vi "报警流程.vi"   [LabVIEW 2016, in "采配水.lvlib"]
uses:
  <vilib>/ptbypt/NI_PtbyPt.lvlib
types:
  T1 = cluster{"低压报警阈值 V":dbl, "低压报警解除阈值 V":dbl, "高温报警阈值 ℃":dbl, "高温报警解除阈值 ℃":dbl, "湿度报警阈值 %":dbl, "湿度报警解除阈值 %":dbl}
  T2 = cluster{"蓄电池电压":dbl, "室温":dbl, "湿度":dbl, "水浸报警":bool, "烟雾报警":bool, "门禁1状态":bool, "门禁2状态":bool}
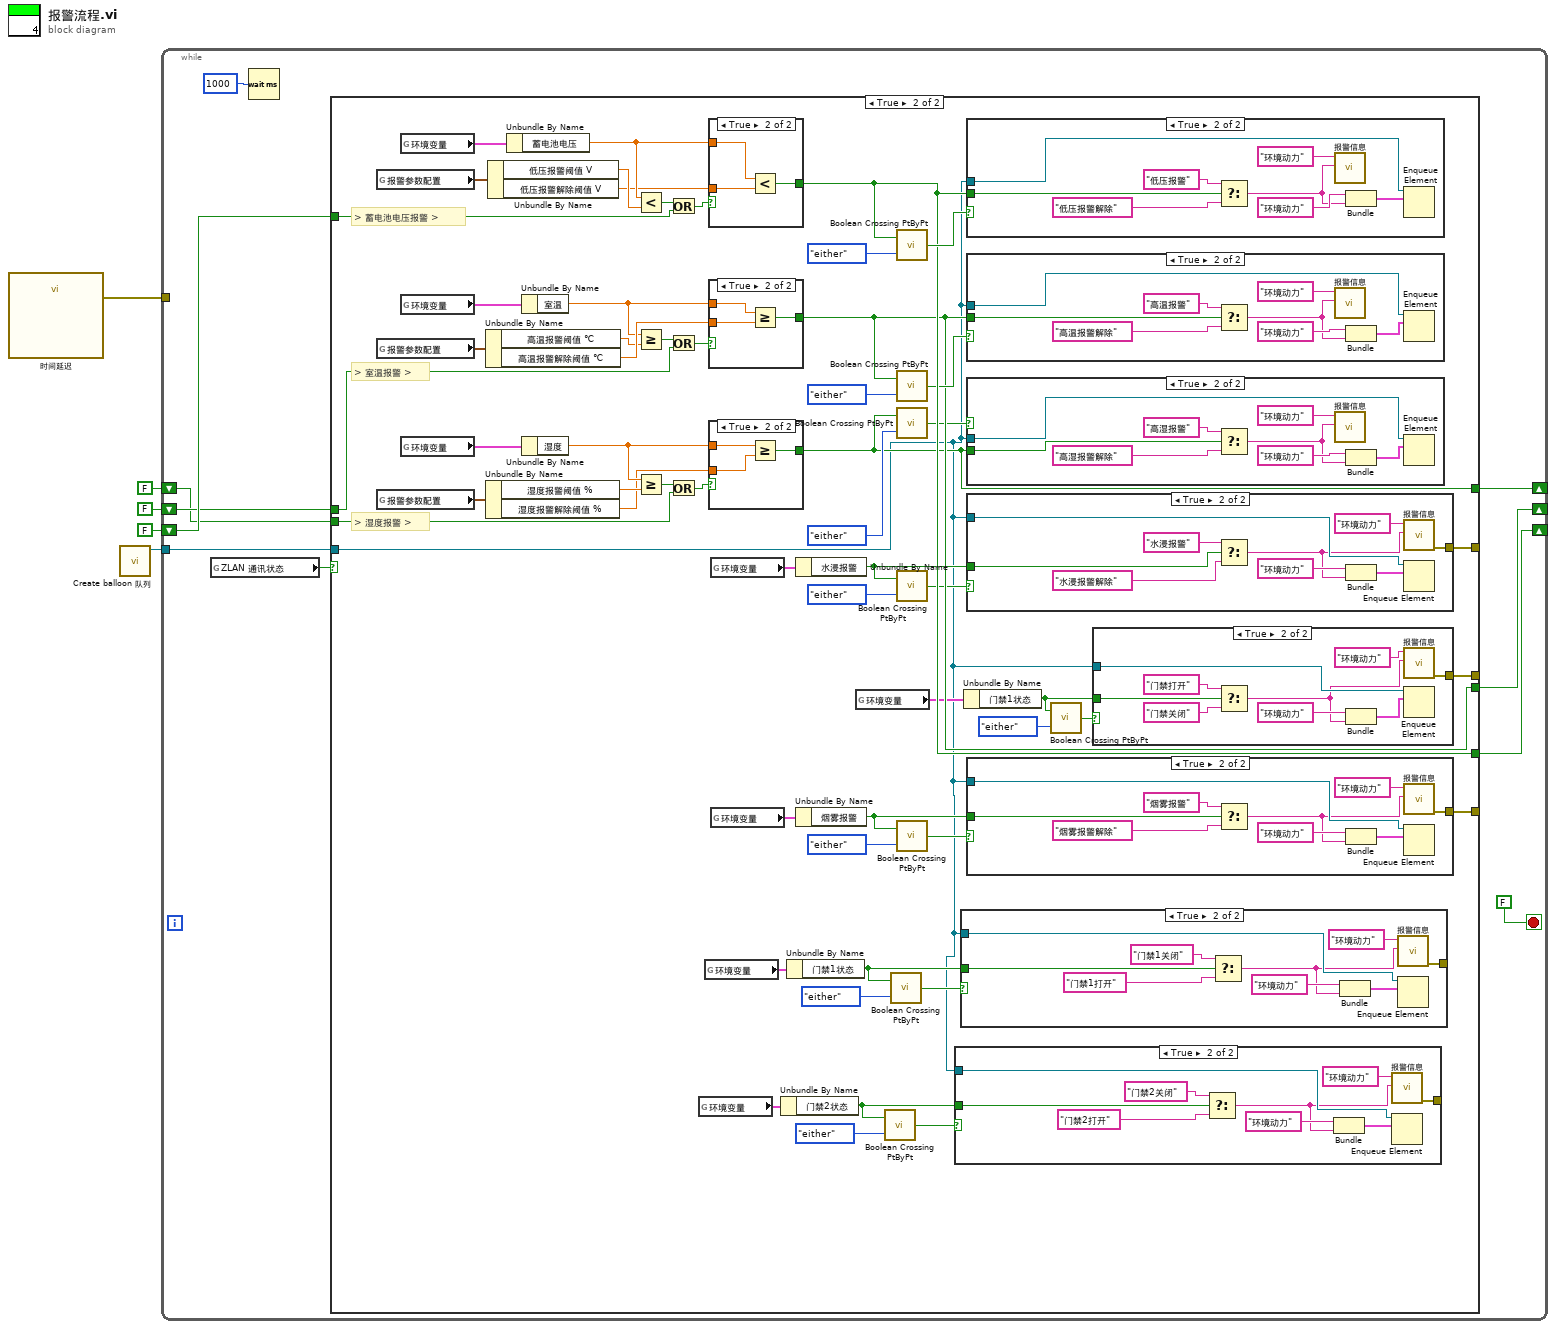
[diagram p0: block diagram]
diagram:
  n1 = call "时间延迟"() -> ("error out"=w1:errorcluster)  [unwired: 11 in]
  n2 = call "Create balloon 队列.vi"() -> ("队列输出"=w5:refnum<queue>)  [unwired: 11 in]
  n3 = while {
    shift-right: [w13] -> _
    shift-left: FALSE -> [w12]
    shift-right: [w10] -> _
    shift-left: FALSE -> [w11]
    shift-right: [w9] -> _
    shift-left: FALSE -> [w8]
    tunnel: w5 -> [w6]
    tunnel: w1 -> [_]
    stop <- FALSE stop-if-true
    n4 = global read "通讯全局变量.vi" "ZLAN 通讯状态"() -> (w7:bool)
    n5 = Wait (ms)(milliseconds to wait=u32 1000 ("等待时间（毫秒）")) -> ()  [unwired: 1 out]
    n6 = case shown="True" w7 {
      tunnel: [_ w46] -> w13
      tunnel: w12 -> [_ w65]
      tunnel: w11 -> [_ w64]
      tunnel: [_ w43] -> w10
      tunnel: [_ w40] -> w9
      tunnel: w8 -> [_ w49]
      tunnel: [_ w35] -> _
      tunnel: [_ w34] -> _
      tunnel: [_ w25] -> _
      tunnel: w6 -> [_ w16]
      frame False {
      }
      frame True {
        # "> 湿度报警 >"
        # "> 室温报警 >"
        # "> 蓄电池电压报警 >"
        n7 = global read "通讯全局变量断电保存.vi" "报警参数配置"() -> (w72:T1)
        n8 = global read "通讯全局变量断电保存.vi" "报警参数配置"() -> (w57:T1)
        n9 = global read "通讯全局变量断电保存.vi" "报警参数配置"() -> (w56:T1)
        n10 = global read "通讯全局变量.vi" "环境变量"() -> (w71:T2)
        n11 = global read "通讯全局变量.vi" "环境变量"() -> (w58:T2)
        n12 = global read "通讯全局变量.vi" "环境变量"() -> (w55:T2)
        n13 = Unbundle By Name(w57) -> ("高温报警阈值 ℃"=w59:dbl, "高温报警解除阈值 ℃"=w62:dbl)
        n14 = Unbundle By Name(w56) -> ("湿度报警阈值 %"=w54:dbl, "湿度报警解除阈值 %"=w51:dbl)
        n15 = Unbundle By Name(w72) -> ("低压报警阈值 V"=w70:dbl, "低压报警解除阈值 V"=w67:dbl)
        n16 = Unbundle By Name(w71) -> ("蓄电池电压"=w68:dbl)
        n17 = Unbundle By Name(w58) -> ("室温"=w61:dbl)
        n18 = Unbundle By Name(w55) -> ("湿度"=w52:dbl)
        n19 = Less?(x=w68, y=w70) -> (x < y?=w69:bool)
        n20 = Greater Or Equal?(x=w61, y=w59) -> (x >= y?=w60:bool)
        n21 = Greater Or Equal?(x=w52, y=w54) -> (x >= y?=w53:bool)
        n22 = Or(x=w69, y=w65) -> (x .or. y?=w66:bool)
        n23 = Or(x=w60, y=w64) -> (x .or. y?=w63:bool)
        n24 = Or(x=w53, y=w49) -> (x .or. y?=w50:bool)
        n25 = global read "通讯全局变量.vi" "环境变量"() -> (w19:T2)
        n26 = global read "通讯全局变量.vi" "环境变量"() -> (w22:T2)
        n27 = case shown="True" w66 {
          tunnel: w68 -> [_ w150]
          tunnel: w67 -> [_ w149]
          tunnel: [_ w148] -> w46
          frame False {
          }
          frame True {
            n28 = Less?(x=w150, y=w149) -> (x < y?=w148:bool)
          }
        }
        n29 = case shown="True" w63 {
          tunnel: w61 -> [_ w147]
          tunnel: w62 -> [_ w146]
          tunnel: [_ w145] -> w43
          frame False {
          }
          frame True {
            n30 = Greater Or Equal?(x=w147, y=w146) -> (x >= y?=w145:bool)
          }
        }
        n31 = case shown="True" w50 {
          tunnel: w52 -> [_ w144]
          tunnel: w51 -> [_ w143]
          tunnel: [_ w142] -> w40
          frame False {
          }
          frame True {
            n32 = Greater Or Equal?(x=w144, y=w143) -> (x >= y?=w142:bool)
          }
        }
        n33 = global read "通讯全局变量.vi" "环境变量"() -> (w37:T2)
        n34 = global read "通讯全局变量.vi" "环境变量"() -> (w32:T2)
        n35 = Unbundle By Name(w19) -> ("门禁2状态"=w20:bool)
        n36 = Unbundle By Name(w22) -> ("门禁1状态"=w21:bool)
        n37 = Unbundle By Name(w37) -> ("水浸报警"=w36:bool)
        n38 = Unbundle By Name(w32) -> ("烟雾报警"=w33:bool)
        n39 = global read "通讯全局变量.vi" "环境变量"() -> (w27:T2)
        n40 = call <vilib>:"Boolean Crossing PtByPt.vi"("direction"=enum16{"either", "false-true", "true-false"}."either", "input"=w20) -> ("crossing"=w18:bool)  [unwired: 1 in]
        n41 = call <vilib>:"Boolean Crossing PtByPt.vi"("direction"=enum16{"either", "false-true", "true-false"}."either", "input"=w21) -> ("crossing"=w23:bool)  [unwired: 1 in]
        n42 = call <vilib>:"Boolean Crossing PtByPt.vi"("direction"=enum16{"either", "false-true", "true-false"}."either", "input"=w46) -> ("crossing"=w47:bool)  [unwired: 1 in]
        n43 = call <vilib>:"Boolean Crossing PtByPt.vi"("direction"=enum16{"either", "false-true", "true-false"}."either", "input"=w43) -> ("crossing"=w44:bool)  [unwired: 1 in]
        n44 = call <vilib>:"Boolean Crossing PtByPt.vi"("direction"=enum16{"either", "false-true", "true-false"}."either", "input"=w40) -> ("crossing"=w42:bool)  [unwired: 1 in]
        n45 = call <vilib>:"Boolean Crossing PtByPt.vi"("direction"=enum16{"either", "false-true", "true-false"}."either", "input"=w36) -> ("crossing"=w38:bool)  [unwired: 1 in]
        n46 = call <vilib>:"Boolean Crossing PtByPt.vi"("direction"=enum16{"either", "false-true", "true-false"}."either", "input"=w33) -> ("crossing"=w31:bool)  [unwired: 1 in]
        n47 = case shown="True" w18 {
          tunnel: w20 -> [_ w80]
          tunnel: [_ w77] -> _
          tunnel: w16 -> [_ w76]
          frame False {
          }
          frame True {
            n48 = Select(t="门禁2关闭" ("设备"), s=w80, f="门禁2打开" ("设备")) -> (s? t:f=w74:string)
            n49 = Bundle("设备"="环境动力", "设备"=w74) -> (w73:cluster{"设备":string, "设备":string})  [unwired: 1 in]
            n50 = call "报警信息.vi"("报警信息"=w74, "设备"="环境动力") -> ("error out"=w77:errorcluster)  [unwired: 9 in]
            n51 = Enqueue Element(queue=w76, element=w73) -> ()  [unwired: 2 in, 3 out]
          }
        }
        n52 = case shown="True" w23 {
          tunnel: w21 -> [_ w89]
          tunnel: [_ w86] -> _
          tunnel: w16 -> [_ w85]
          frame False {
          }
          frame True {
            n53 = Select(t="门禁1关闭" ("设备"), s=w89, f="门禁1打开" ("设备")) -> (s? t:f=w83:string)
            n54 = Bundle("设备"="环境动力", "设备"=w83) -> (w82:cluster{"设备":string, "设备":string})  [unwired: 1 in]
            n55 = call "报警信息.vi"("报警信息"=w83, "设备"="环境动力") -> ("error out"=w86:errorcluster)  [unwired: 9 in]
            n56 = Enqueue Element(queue=w85, element=w82) -> ()  [unwired: 2 in, 3 out]
          }
        }
        n57 = Unbundle By Name(w27) -> ("门禁1状态"=w26:bool)
        n58 = case shown="True" w47 {
          tunnel: w46 -> [_ w140]
          tunnel: w16 -> [_ w135]
          frame False {
          }
          frame True {
            n59 = Select(t="低压报警" ("设备"), s=w140, f="低压报警解除" ("设备")) -> (s? t:f=w134:string)
            n60 = call "报警信息.vi"("报警信息"=w134, "设备"="环境动力") -> ()  [unwired: 9 in, 1 out]
            n61 = Bundle("设备"="环境动力", "设备"=w134) -> (w136:cluster{"设备":string, "设备":string})  [unwired: 1 in]
            n62 = Enqueue Element(queue=w135, element=w136) -> ()  [unwired: 2 in, 3 out]
          }
        }
        n63 = case shown="True" w44 {
          tunnel: w43 -> [_ w132]
          tunnel: w16 -> [_ w127]
          frame False {
          }
          frame True {
            n64 = Select(t="高温报警" ("设备"), s=w132, f="高温报警解除" ("设备")) -> (s? t:f=w126:string)
            n65 = call "报警信息.vi"("报警信息"=w126, "设备"="环境动力") -> ()  [unwired: 9 in, 1 out]
            n66 = Bundle("设备"="环境动力", "设备"=w126) -> (w128:cluster{"设备":string, "设备":string})  [unwired: 1 in]
            n67 = Enqueue Element(queue=w127, element=w128) -> ()  [unwired: 2 in, 3 out]
          }
        }
        n68 = case shown="True" w42 {
          tunnel: w40 -> [_ w124]
          tunnel: w16 -> [_ w119]
          frame False {
          }
          frame True {
            n69 = Select(t="高湿报警" ("设备"), s=w124, f="高湿报警解除" ("设备")) -> (s? t:f=w118:string)
            n70 = call "报警信息.vi"("报警信息"=w118, "设备"="环境动力") -> ()  [unwired: 9 in, 1 out]
            n71 = Bundle("设备"="环境动力", "设备"=w118) -> (w121:cluster{"设备":string, "设备":string})  [unwired: 1 in]
            n72 = Enqueue Element(queue=w119, element=w121) -> ()  [unwired: 2 in, 3 out]
          }
        }
        n73 = case shown="True" w38 {
          tunnel: w36 -> [_ w116]
          tunnel: [_ w113] -> w35
          tunnel: w16 -> [_ w110]
          frame False {
          }
          frame True {
            n74 = Select(t="水浸报警" ("设备"), s=w116, f="水浸报警解除" ("设备")) -> (s? t:f=w109:string)
            n75 = Bundle("设备"="环境动力", "设备"=w109) -> (w112:cluster{"设备":string, "设备":string})  [unwired: 1 in]
            n76 = call "报警信息.vi"("报警信息"=w109, "设备"="环境动力") -> ("error out"=w113:errorcluster)  [unwired: 9 in]
            n77 = Enqueue Element(queue=w110, element=w112) -> ()  [unwired: 2 in, 3 out]
          }
        }
        n78 = case shown="True" w31 {
          tunnel: w33 -> [_ w107]
          tunnel: [_ w104] -> w34
          tunnel: w16 -> [_ w103]
          frame False {
          }
          frame True {
            n79 = Select(t="烟雾报警" ("设备"), s=w107, f="烟雾报警解除" ("设备")) -> (s? t:f=w101:string)
            n80 = Bundle("设备"="环境动力", "设备"=w101) -> (w100:cluster{"设备":string, "设备":string})  [unwired: 1 in]
            n81 = call "报警信息.vi"("报警信息"=w101, "设备"="环境动力") -> ("error out"=w104:errorcluster)  [unwired: 9 in]
            n82 = Enqueue Element(queue=w103, element=w100) -> ()  [unwired: 2 in, 3 out]
          }
        }
        n83 = call <vilib>:"Boolean Crossing PtByPt.vi"("direction"=enum16{"either", "false-true", "true-false"}."either", "input"=w26) -> ("crossing"=w28:bool)  [unwired: 1 in]
        n84 = case shown="True" w28 {
          tunnel: w26 -> [_ w98]
          tunnel: [_ w95] -> w25
          tunnel: w16 -> [_ w93]
          frame False {
          }
          frame True {
            n85 = Select(t="门禁打开" ("设备"), s=w98, f="门禁关闭" ("设备")) -> (s? t:f=w92:string)
            n86 = Bundle("设备"="环境动力", "设备"=w92) -> (w91:cluster{"设备":string, "设备":string})  [unwired: 1 in]
            n87 = call "报警信息.vi"("报警信息"=w92, "设备"="环境动力") -> ("error out"=w95:errorcluster)  [unwired: 9 in]
            n88 = Enqueue Element(queue=w93, element=w91) -> ()  [unwired: 2 in, 3 out]
          }
        }
      }
    }
  }
